vi "unpair modules.vi"(6 "paired engine in":refnum<class "engine configuration.lvclass">, 8 "error in":errorcluster, 9 "engine configuration in":refnum<class "engine configuration.lvclass">, 10 "module to unpair":refnum<class "TEC editor node.lvclass">, 11 "UDP Broadcast Editor Node in":refnum<class "TEC editor node.lvclass">) -> (0 "error out":errorcluster, 1 "engine configuration out":refnum<class "engine configuration.lvclass">, 2 "unpaired module":refnum<class "TEC editor node.lvclass">, 3 "UDP Broadcast Editor Node out":refnum<class "TEC editor node.lvclass">, 4 "paired engine out":refnum<class "engine configuration.lvclass">)   [LabVIEW 2013, in "TEC editor node.lvclass"]
uses:
  TEC editor node.lvclass
  <vilib>/NI/Module Execution Interface/Engine Configuration/engine configuration.lvclass
  TEC editor node.lvclass/TEC editor node.ctl
  <vilib>/NI/Configuration Framework/serializable configuration/NISE_CEF_serializable configuration.lvclass
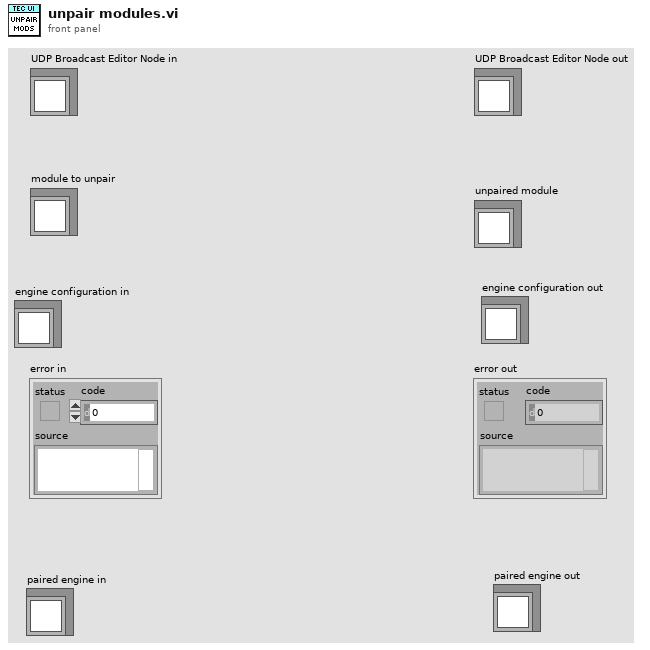
[diagram p1: front panel]
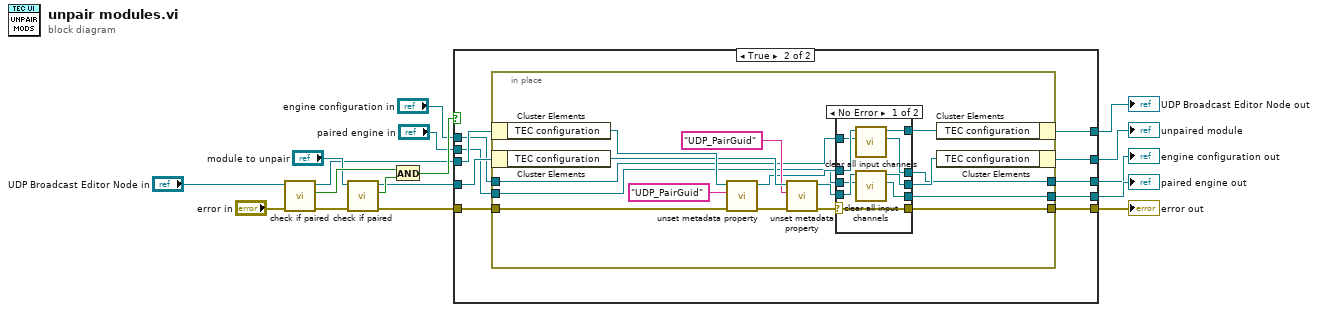
[diagram p0: block diagram]
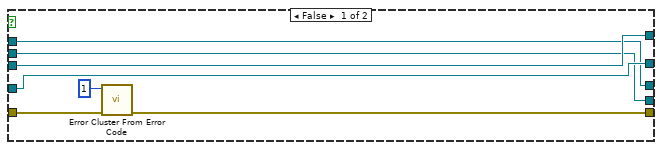
[diagram p2: hidden frame]
diagram:
  n1 = call "check if paired.vi"("error in"="error in", "UDP Broadcast Editor Node in"="UDP Broadcast Editor Node in") -> ("error out"=w12:errorcluster, "paired"=w16:bool, "UDP Broadcast Editor Node out"=w7:refnum<class "TEC editor node.lvclass">)  [unwired: 7 in]
  n2 = call "check if paired.vi"("error in"=w12, "UDP Broadcast Editor Node in"="module to unpair") -> ("error out"=w10:errorcluster, "paired"=w17:bool, "UDP Broadcast Editor Node out"=w5:refnum<class "TEC editor node.lvclass">)  [unwired: 7 in]
  n3 = And(x=w16, y=w17) -> (x .and. y?=w11:bool)
  n4 = case shown="True" w11 {
    tunnel: w10 -> [w23 w32]
    tunnel: [w22 w28] -> w9
    tunnel: [w21 w26] -> w8
    tunnel: w7 -> [w21 w34]
    tunnel: [w20 w27] -> w6
    tunnel: w5 -> [w20 w33]
    tunnel: "paired engine in" -> [w19 w30]
    tunnel: [w19 w29] -> w3
    tunnel: "engine configuration in" -> [w18 w31]
    tunnel: [w18 w25] -> w1
    frame False {
      n5 = call <vilib>:"Error Cluster From Error Code.vi"("error in (no error)"=w23, "error code (0)"=1) -> ("error out"=w22:errorcluster)  [unwired: 7 in]
    }
    frame True {
      n6 = in-place {
        in-place-border: [w44] -> w28
        in-place-border: w32 -> [w39]
        in-place-border: w31 -> [w38]
        in-place-border: w30 -> [w37]
        in-place-border: [w36] -> w29
        in-place-border: [w35] -> w25
        n7 = in-place-cluster #1(w34) -> ("TEC configuration"=w50:refnum<class "TEC configuration.lvclass">)
        n8 = in-place-cluster #2(w33) -> ("TEC configuration"=w49:refnum<class "TEC configuration.lvclass">)
        n9 = call <vilib>:"unset metadata property.vi"("error in"=w39, "key"="UDP_PairGuid", "configuration in"=w50) -> ("error out"=w46:errorcluster, "configuration out"=w40:refnum<class "TEC configuration.lvclass">)  [unwired: 7 in]
        n10 = call <vilib>:"unset metadata property.vi"("error in"=w46, "key"="UDP_PairGuid", "configuration in"=w49) -> ("error out"=w45:errorcluster, "configuration out"=w43:refnum<class "TEC configuration.lvclass">)  [unwired: 7 in]
        n11 = case shown="No Error" w45 {
          selector: w45 -> [w55 w64]
          tunnel: [w55 w64] -> w44
          tunnel: w43 -> [w59 w63]
          tunnel: [w56 w63] -> w42
          tunnel: [w57 w62] -> w41
          tunnel: w40 -> [w58 w62]
          tunnel: w38 -> [w54 w61]
          tunnel: w37 -> [w53 w60]
          tunnel: [w52 w60] -> w36
          tunnel: [w51 w61] -> w35
          frame No Error {
            n12 = call "clear all input channels.vi"("engine configuration in"=w54, "TEC configuration in"=w58) -> ("engine configuration out"=w51:refnum<class "engine configuration.lvclass">, "TEC configuration out"=w57:refnum<class "TEC configuration.lvclass">)  [unwired: 8 in]
            n13 = call "clear all input channels.vi"("engine configuration in"=w53, "TEC configuration in"=w59) -> ("engine configuration out"=w52:refnum<class "engine configuration.lvclass">, "TEC configuration out"=w56:refnum<class "TEC configuration.lvclass">)  [unwired: 8 in]
          }
          frame Error {
          }
        }
        n14 = in-place-cluster #1("TEC configuration"=w41) -> (w26:refnum<class "TEC editor node.lvclass">)
        n15 = in-place-cluster #2("TEC configuration"=w42) -> (w27:refnum<class "TEC editor node.lvclass">)
      }
    }
  }
  "error out" <- w9
  "UDP Broadcast Editor Node out" <- w8
  "unpaired module" <- w6
  "engine configuration out" <- w1
  "paired engine out" <- w3
